vi "Do.vi"(8 "error in (no error)":errorcluster, 10 "Actor in":refnum<class "Actor.lvclass">, 11 "Poll Msg":refnum<class "Ping Msg.lvclass">) -> (0 "error out":errorcluster, 2 "Actor out":refnum<class "Actor.lvclass">)   [LabVIEW 2018, in "Monitored Actor.lvlib" / "Ping Msg.lvclass"]
doc: "(<B>Filename</B>: Actor Framework.lvlib:Message.lvclass:Do.vi)\n\nDefines what a message does when it is received by an actor. Generally, a message instructs an actor to invoke one of its methods.\n\nBy default, this method does nothing. A child class must override it to define behavior. Create a child class by using the Actor Framework Message Maker dialog box."
uses:
  Ping Msg.lvclass
  <vilib>/ActorFramework/Actor/Actor.lvclass
  Actor/Monitored Actor.lvclass
  C:/Program Files (x86)/National Instruments/LabVIEW 2018/vi.lib/ActorFramework/Actor/Actor.lvclass
  Actor/Monitored Actor.lvclass/Monitored Actor.ctl
  Ping Msg.lvclass/Ping Msg.ctl
  Actor Monitor/Actor Monitor Messages/Ping Response Msg/Ping Response Msg.lvclass/Ping Response Msg.ctl
  <vilib>/ActorFramework/Message Enqueuer/Message Enqueuer.lvclass/Message Enqueuer.ctl
  <vilib>/ActorFramework/Message Enqueuer/Enqueue.vi
  Actor Monitor/Actor Monitor Messages/Ping Response Msg/Ping Response Msg.lvclass
  C:/Program Files (x86)/National Instruments/LabVIEW 2018/vi.lib/ActorFramework/Message/Message.lvclass
  <vilib>/ActorFramework/Message Priority Queue/Priority Enqueue.vi
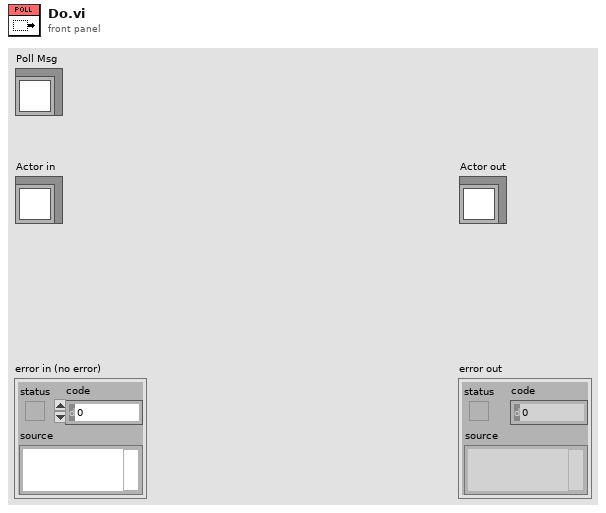
[diagram p1: front panel]
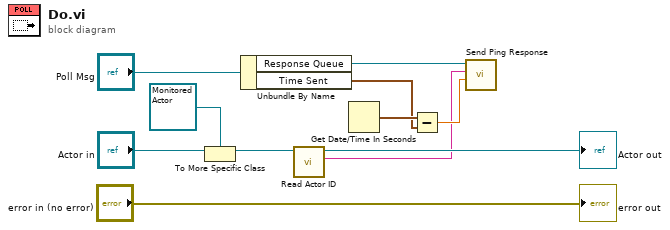
[diagram p0: block diagram]
diagram:
  n1 = To More Specific Class(target class=refnum<class "Monitored Actor.lvclass"> refnum ("Monitored Actor.lvlib:Monitored Actor.lvclass"), reference="Actor in") -> (specific class reference=w7:refnum<class "Monitored Actor.lvclass">)  [unwired: 1 in, 1 out]
  n2 = Unbundle By Name("Poll Msg") -> ("Response Queue"=w5:refnum<class "Message Enqueuer.lvclass">, "Time Sent"=w1:timestamp)
  n3 = call "Read Actor ID.vi"("Monitored Actor in"=w7) -> ("Actor ID"=w3:string, "Monitored Actor out"=→"Actor out":refnum<class "Monitored Actor.lvclass">)  [unwired: 9 in]
  n4 = Get Date/Time In Seconds() -> (seconds since 1Jan1904=w2:timestamp)
  n5 = Subtract(x=w2, y=w1) -> (x-y=w4:dbl)
  n6 = call "Send Ping Response.vi"("Seconds to Respond"=w4, "Actor Core Name"=w3, "Message Enqueuer"=w5) -> ()  [unwired: 7 in, 2 out]
  "error out" <- "error in (no error)"
